vi "Agilent SNA Set Trigger Mode (SWP).vi"(6 "Channel":i8=1 min=1 max=99 step=1, 7 "Agilent SNA":T1, 8 "error in (no error)":errorcluster, 10 "Trigger Mode":T2, 11 "VISA Resource Names":T3) -> (0 "error out":errorcluster, 3 "dup VISA Resource Names":T3)   [LabVIEW 2011]
doc: "This VI for the HP8753B Network Analyzers reads the stimulus values. Except when performing log sweeps and freq list sweeps, this VI uses the start and stop values and the number of points to calcuate the stimulus values."
uses:
  TypeDefs/Agilent SNA Trigger Mode.ctl
  TypeDefs/Agilent SNA Instrument Info.ctl
  TypeDefs/Agilent SNA VISA.ctl
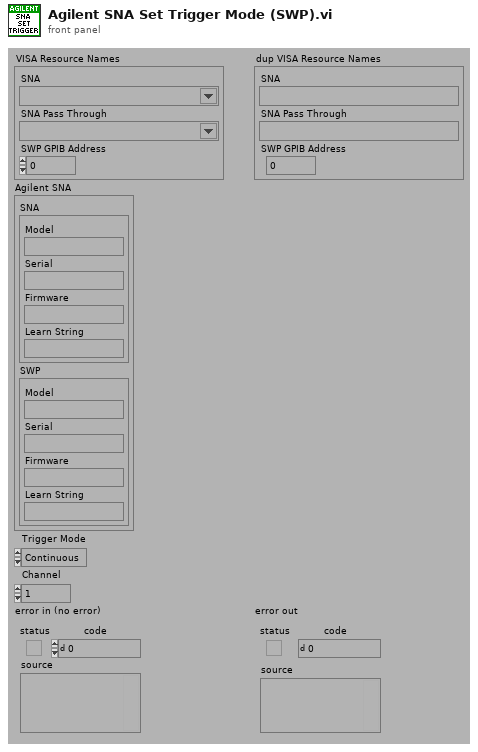
[diagram p1: front panel]
types:
  T1 = typedef "Agilent SNA Instrument Info.ctl" = cluster{"SNA":cluster{"Model":string, "Serial":string, "Firmware":string, "Learn String":string}, "SWP":cluster{"Model":string, "Serial":string, "Firmware":string, "Learn String":string}}
  T2 = typedef "Agilent SNA Trigger Mode.ctl" = enum16{"Continuous", "Hold", "Single"}
  T3 = typedef "Agilent SNA VISA.ctl" = cluster{"SNA":refnum<visa-resource-name>, "SNA Pass Through":refnum<visa-resource-name>, "SWP GPIB Address":i32}
  T4 = typedef "Agilent SNA Model.ctl" = enum16{"Not Supported", "8757X"}
  T5 = typedef "Agilent SNA SWP Model.ctl" = enum16{"Not Supported", "836XXX", "8375XX", "E82X7D"}
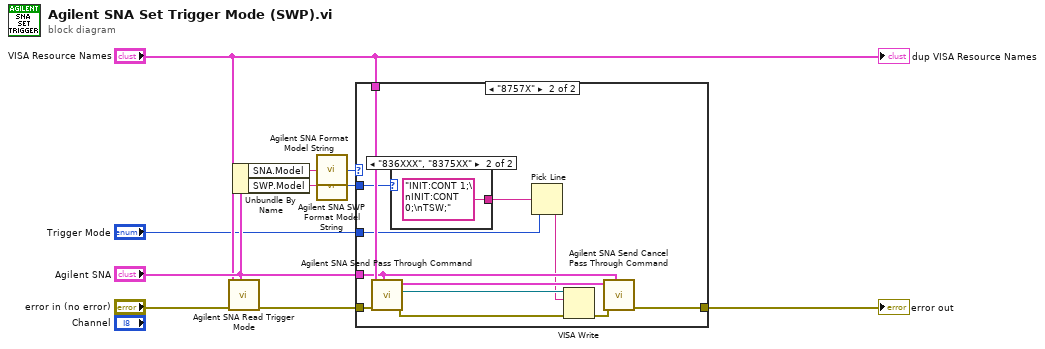
[diagram p0: block diagram]
diagram:
  n1 = call "Agilent SNA Read Trigger Mode.vi"("Agilent SNA & SWP"="Agilent SNA", "error in (no error)"="error in (no error)", "VISA Resource Names"="VISA Resource Names") -> ("error out"=w6:errorcluster)  [unwired: 6 in, 2 out]
  n2 = Unbundle By Name("Agilent SNA") -> ("SNA.Model"=w10:string, "SWP.Model"=w8:string)
  n3 = call "Agilent SNA Format Model String.vi"("Model String"=w10) -> ("Model"=w9:T4)
  n4 = call "Agilent SNA SWP Format Model String.vi"("Model String"=w8) -> ("Model"=w7:T5)
  n5 = case shown="\"8757X\"" w9 {
    tunnel: w6 -> [w11 w23]
    tunnel: [w11 w19] -> w3
    tunnel: "Agilent SNA" -> [_ w18]
    tunnel: "VISA Resource Names" -> [_ w20]
    tunnel: w7 -> [_ w16]
    tunnel: "Trigger Mode" -> [_ w12]
    frame "Not Supported" {
    }
    frame "8757X" {
      n6 = call "Agilent SNA Send Pass Through Command.vi"("Agilent SNA & SWP"=w18, "error in (no error)"=w23, "VISA Resource Names"=w20) -> ("error out"=w22:errorcluster, "SNA Pass Through"=w21:refnum<visa-resource-name>, "dup VISA Resource Names"=w17:T3)  [unwired: 6 in]
      n7 = case shown="\"836XXX\", \"8375XX\"" w16 {
        tunnel: [_ "INIT:CONT 1;\nINIT:CONT 0;\nTSW;"] -> w13
        frame "Not Supported" {
        }
        frame "836XXX", "8375XX" {
        }
      }
      n8 = Pick Line(multi-line string=w13, line index=w12) -> (output string=w14:string)  [unwired: 1 in]
      n9 = VISA Write(VISA resource name=w21, write buffer=w14, error in (no error)=w22) -> (error out=w15:errorcluster)  [unwired: 2 out]
      n10 = call "Agilent SNA Send Cancel Pass Through Command.vi"("Agilent SNA & SWP"=w18, "error in (no error)"=w15, "VISA Resource Names"=w17) -> ("error out"=w19:errorcluster)  [unwired: 7 in, 1 out]
    }
  }
  "error out" <- w3
  "dup VISA Resource Names" <- "VISA Resource Names"
